vi "Configure Measurement Source.vi"(8 "error in (no error)":errorcluster, 9 "Source 2 (21: None)":u16(ring)=21 items=["Channel 1", "Channel 2", "Channel 3", "Channel 4", "DIG 0", "DIG 1", "DIG 2", "DIG 3", "DIG 4", "DIG 5", "DIG 6", "DIG 7", "DIG 8", "DIG 9", "DIG 10", "DIG 11", "DIG 12", "DIG 13", "DIG 14", "DIG 15", "Math", "None"], 10 "Source 1 (0: Channel 1)":u16(ring) items=["Channel 1", "Channel 2", "Channel 3", "Channel 4", "DIG 0", "DIG 1", "DIG 2", "DIG 3", "DIG 4", "DIG 5", "DIG 6", "DIG 7", "DIG 8", "DIG 9", "DIG 10", "DIG 11", "DIG 12", "DIG 13", "DIG 14", "DIG 15", "Math"], 11 "VISA resource name":refnum<visa-resource-name>) -> (0 "error out":errorcluster, 3 "VISA resource name out":refnum<visa-resource-name>)   [LabVIEW 2017, in "Agilent 6000 Series.lvlib"]
doc: "This VI configures the properties that control the measurement source. These properties are the source 1 and source 2.\n\n<B>Note:</B>\n\n(1) This VI has been obsoleted from the driver and is included for compatibility with existing applications. New applications should use the <B>Fetch Measurement</B> and <B>Read Measurement</B> VIs."
uses:
  <instrlib>/Agilent 6000 Series/Agilent 6000 Series.lvlib
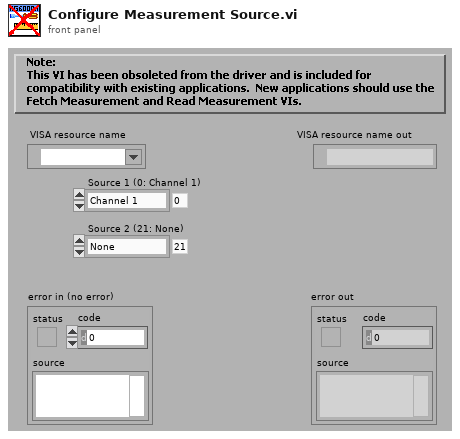
[diagram p1: front panel]
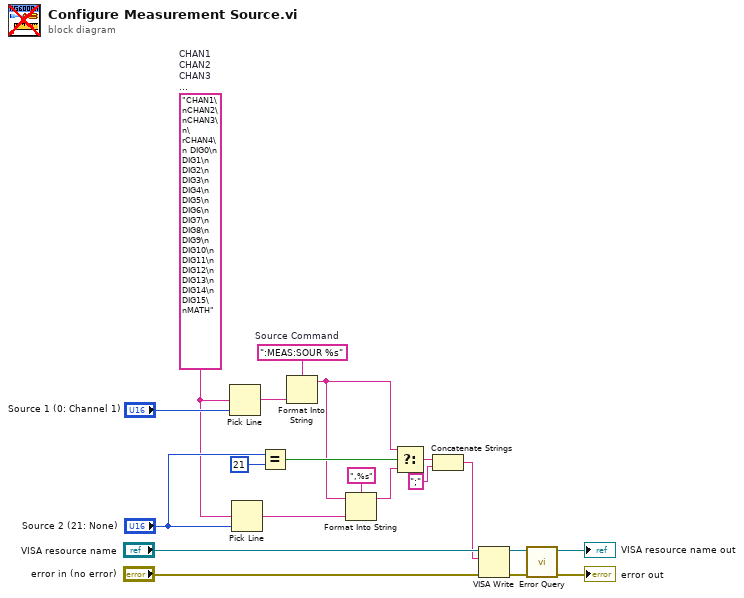
[diagram p0: block diagram]
diagram:
  w4 = "CHAN1\nCHAN2\nCHAN3\n\rCHAN4\n DIG0\n DIG1\n DIG2\n DIG3\n DIG4\n DIG5\n DIG6\n DIG7\n DIG8\n DIG9\n DIG10\n DIG11\n DIG12\n DIG13\n DIG14\n DIG15\nMATH"  # CHAN1 CHAN2 CHAN3  CHAN4  DIG0  DIG1  DIG2  DIG3  DIG4  DIG5  DIG6  DIG7  DIG8  DIG9  DIG10  DIG11  DIG12  DIG13  DIG14  DIG15 MATH
  w14 = ":MEAS:SOUR %s"  # Source Command
  n1 = Pick Line(multi-line string=w4, line index="Source 1 (0: Channel 1)") -> (output string=w13:string)  [unwired: 1 in]
  n2 = Pick Line(multi-line string=w4, line index="Source 2 (21: None)") -> (output string=w7:string)  [unwired: 1 in]
  n3 = Equal?(x="Source 2 (21: None)", y=u16 21) -> (x = y?=w11:bool)
  n4 = Format Into String(format string=w14, w13) -> (resulting string=w5:string)  [unwired: 2 in, 1 out]
  n5 = Format Into String(format string=",%s", initial string=w5, w7) -> (resulting string=w6:string)  [unwired: 1 in, 1 out]
  n6 = Select(t=w5, s=w11, f=w6) -> (s? t:f=w3:string)
  n7 = Concatenate Strings(w3, ";" ("string")) -> (w1:string)
  n8 = VISA Write(VISA resource name="VISA resource name", write buffer=w1, error in (no error)="error in (no error)") -> (VISA resource name out=w16:refnum<visa-resource-name>, error out=w15:errorcluster)  [unwired: 1 out]
  n9 = call <instrlib>:"Error Query.vi"("error in (no error)"=w15, "VISA resource name"=w16) -> ("error out"=→"error out":errorcluster, "VISA resource name out"=→"VISA resource name out":refnum<visa-resource-name>)  [unwired: 6 in, 2 out]
